vi "ProcImage.vi"(6 "Array Data In":i16[][][](array[numeric]), 8 "Att Array (dB)":sgl[](array[numeric])) -> (0 "Syth App Data":i16[][][](array[numeric]), 2 "Att (dB)":sgl[](array[numeric]), 4 "Focal lengths":sgl[](array[numeric])=[0.0085, 0.009, 0.0095, 0.01, 0.0105, 0.011, 0.0115, 0.012, 0.0125, 0.013, 0.0135, 0.014, 0.0145, 0.015])   [LabVIEW 2022 SP3]
uses:
  ScanningControl/Motion Controllers/-MotionRoutines/MotionGlobals.vi
  <vilib>/Analysis/NI_AALBase.lvlib
panel:
  in  "Case Constant\n(See Context Help)":bool
  out "Waveform Graph":i16[](graph)
  in  "F- zones":i16=13
  out "Synth App Image":i16[][](graph)
  in  "Radii":sgl[](array[numeric])=[0.0, 0.00132, 0.00142, 0.0019, 0.002, 0.00236, 0.00245, 0.00275, 0.00285, 0.0031]
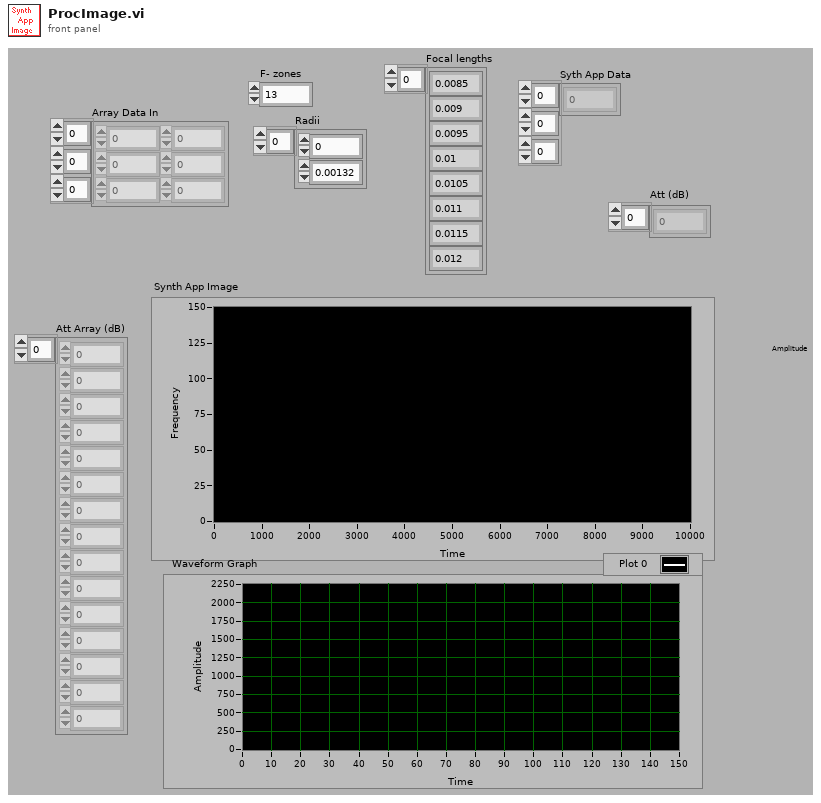
[diagram p1: front panel]
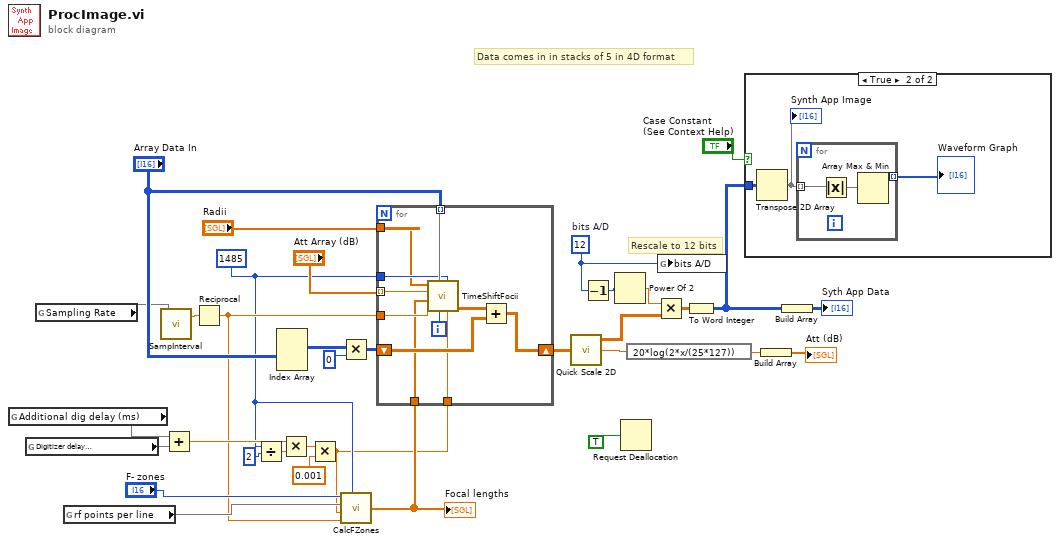
[diagram p0: block diagram]
diagram:
  w17 = 12  # bits A/D
  w4 = 1485
  # "Data comes in in stacks of 5 in 4D format"
  # "Rescale to 12 bits"
  n1 = global read "MotionGlobals.vi" "Additional dig delay (ms)"() -> (w14)
  n2 = global read "MotionGlobals.vi" "Digitizer delay\n (ms)"() -> (w13)
  n3 = global read "MotionGlobals.vi" "Sampling Rate"() -> (w22)
  n4 = global read "MotionGlobals.vi" "rf points per line"() -> (w8)
  n5 = call "SampInterval.vi"("Sampling Rate"=w22) -> ("time (s)"=w6:dbl)  [unwired: 1 in, 1 out]
  n6 = Add(x=w14, y=w13) -> (x+y=w7:dbl)
  n7 = Reciprocal(x=w6) -> (1/x=w5:dbl)
  n8 = Divide(x=w4, y=2) -> (x/y=w23:dbl)
  n9 = Index Array(array="Array Data In") -> (element=w31:i16[][])  [unwired: 3 in]
  n10 = Multiply(x=w7, y=w23) -> (x*y=w16:dbl)
  n11 = Multiply(x=w16, y=0.001) -> (x*y=w1:dbl)
  n12 = Multiply(x=w31, y=0) -> (x*y=w32:i32[][])
  n13 = call "CalcFZones.vi"("F- zones"="F- zones", "# rf points per line"=w8, "delay"=w1, "Sampling Rate"=w5, "c (m/s)"=w4) -> ("Array"=w10:dbl[])
  "Focal lengths" <- w10
  n14 = for {
    tunnel: "Radii" -> [w35]
    tunnel: w5 -> [w45]
    shift-right: [w44] -> w20
    shift-left: w32 -> [w43]
    tunnel: "Array Data In" -> [w42] mode=indexing
    tunnel: "Att Array (dB)" -> [w41] mode=indexing
    tunnel: w1 -> [w38]
    tunnel: w10 -> [w37]
    tunnel: w4 -> [w36]
    i -> [w39]
    n15 = call "TimeShiftFocii.vi"("delay (mm)"=w38, "c (m/s)"=w36, "File index number"=w39, "Array data"=w42, "Sampling Rate (s)"=w45, "Focal lengths (m)"=w37, "attn_dB"=w41, "Radii (m)"=w35) -> ("Synth App Out"=w40:sgl[][])  [unwired: 3 in]
    n16 = Add(x=w40, y=w43) -> (x+y=w44:sgl[][])
  }
  n17 = call <vilib>:"Quick Scale 2D.vi"("X"=w20) -> ("Yij=Xij/Max|X|"=w12:dbl[][], "max|X|"=w28:dbl)  [unwired: 1 out]
  n18 = Decrement(x=w17) -> (x-1=w19:i32)
  n19 = Power Of 2(x=w19) -> (2^x=w18:dbl)
  n20 = Request Deallocation(TRUE) -> ()
  n21 = expression code="20*log(2*x/(25*127))"(w28) -> (w29:dbl)
  n22 = Multiply(x=w18, y=w12) -> (x*y=w27:dbl[][])
  n23 = global write "MotionGlobals.vi" "bits A/D"(w17) -> ()
  n24 = To Word Integer(number=w27) -> (16bit integer=w11:i16[][])
  n25 = case shown="True" "Case Constant\n(See Context Help)" {
    tunnel: w11 -> [_ w46]
    frame False {
    }
    frame True {
      n26 = Transpose 2D Array(2D array=w46) -> (transposed array=w48:i16[][])
      "Synth App Image" <- w48
      n27 = for {
        tunnel: w48 -> [w51] mode=indexing
        tunnel: [w50] -> w47 mode=indexing
        n28 = Absolute Value(x=w51) -> (abs(x)=w49:i16[])
        n29 = Array Max & Min(array=w49) -> (max value=w50:i16)  [unwired: 3 out]
      }
      "Waveform Graph" <- w47
    }
  }
  n30 = Build Array(w29) -> (→"Att (dB)":dbl[])
  n31 = Build Array(w11) -> (→"Syth App Data":i16[][][])
